vi "MaquinaDispensadora.vi"() -> ()   [LabVIEW 2020]
uses:
  Control 1.ctl
panel:
  out "Numeric":dbl
  out "Boolean":bool
  in  "stop":bool
  out "Cambio":dbl
  in  "Estado compra":string
  out "Total":dbl
  out "Precio":dbl
  in  "Moneda":cluster{"$ 10":bool, "$ 20":bool}
  in  "Productos":T1
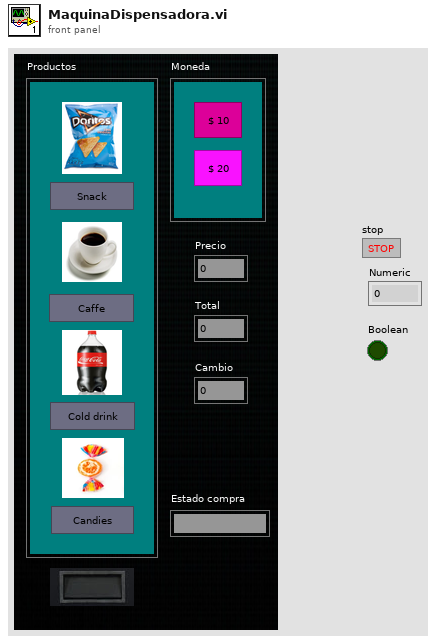
[diagram p1: front panel]
types:
  T1 = cluster{"Snack":bool, "Caffe":bool, " Cold drink":bool, "Candies":bool}
  T2 = typedef "Control 1.ctl" = enum16{"Return Change", "Selecto Product", "Add Money", "Waiting", "Start-UP", "Dispense Product"}
  T3 = cluster{"Cherry Rush":bool, "Lime Fizz":bool, "Orange Blast":bool, "Mr. Fizzle":bool}
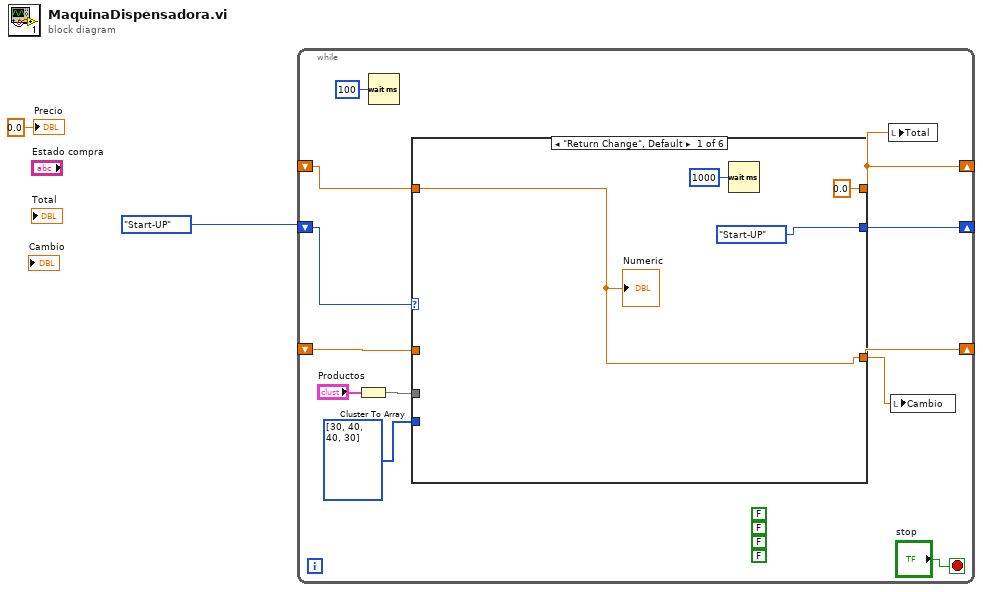
[diagram p0: block diagram]
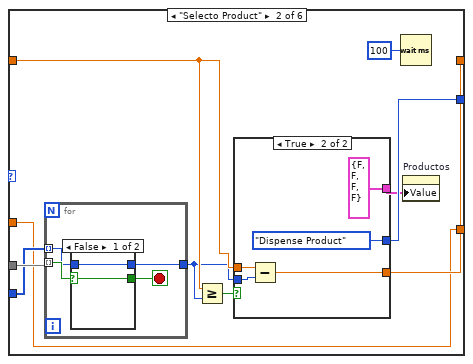
[diagram p2: hidden frame]
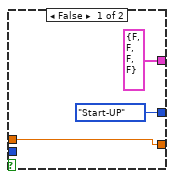
[diagram p3: hidden frame]
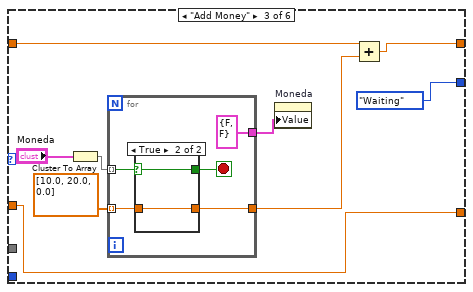
[diagram p5: hidden frame]
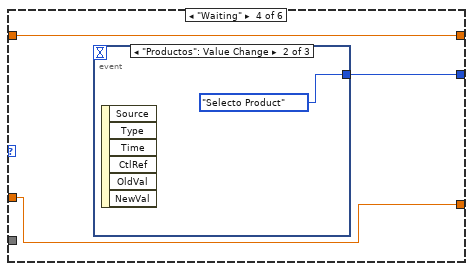
[diagram p7: hidden frame]
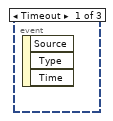
[diagram p8: hidden frame]
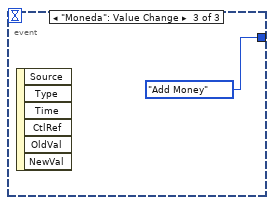
[diagram p9: hidden frame]
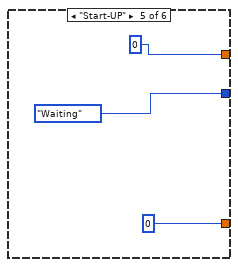
[diagram p10: hidden frame]
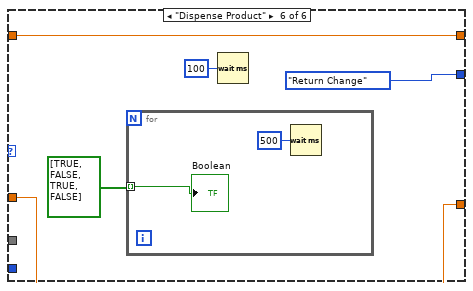
[diagram p11: hidden frame]
diagram:
  n1 = while {
    shift-right: [w9] -> _
    shift-left: Control_1."Start-UP" -> [w11]
    shift-right: [w5] -> _
    shift-left: _ -> [w6]
    shift-right: [w4] -> _
    shift-left: _ -> [w10]
    stop <- "stop" stop-if-true
    (unwired) FALSE ("Mr. Fizzle")
    (unwired) FALSE ("Orange Blast")
    (unwired) FALSE ("Lime Fizz")
    (unwired) FALSE ("Cherry Rush")
    n2 = Cluster To Array(cluster="Productos") -> (array=w8:bool[])
    n3 = Wait (ms)(milliseconds to wait=u32 100) -> ()  [unwired: 1 out]
    n4 = case shown="\"Return Change\", Default" w11 {
      tunnel: [0.0 w22 w48 w63 0 w71] -> w5
      tunnel: [w15 w18 w44 w64 0 w72] -> w4
      tunnel: w10 -> [_ w18 w44 w64 _ w72]
      tunnel: [Control_1."Start-UP" w21 Control_1."Waiting" w62 Control_1."Waiting" Control_1."Return Change"] -> w9
      tunnel: w8 -> [_ w27 _ _ _ _]
      tunnel: i32[] [30, 40, 40, 30] -> [_ w26 _ _ _ _]
      tunnel: w6 -> [w15 w24 w47 w63 _ w71]
      frame "Return Change", Default {
        n5 = Wait (ms)(milliseconds to wait=u32 1000) -> ()  [unwired: 1 out]
        "Numeric" <- w15
      }
      frame "Selecto Product" {
        n6 = for {
          tunnel: w27 -> [w39] mode=indexing
          tunnel: w26 -> [w37] mode=indexing
          tunnel: [w36] -> w23
          stop <- w38 stop-if-true
          n7 = case shown="False" w39 {
            selector: w39 -> [w41 w43]
            tunnel: [w41 w43] -> w38
            tunnel: w37 -> [w40 w42]
            tunnel: [w40 w42] -> w36
            frame False {
            }
            frame True {
            }
          }
        }
        n8 = Greater Or Equal?(x=w24, y=w23) -> (x >= y?=w25:bool)
        n9 = case shown="True" w25 {
          tunnel: w24 -> [w30 w35]
          tunnel: w23 -> [_ w34]
          tunnel: [w30 w33] -> w22
          tunnel: [Control_1."Start-UP" Control_1."Dispense Product"] -> w21
          tunnel: [T3 {"Cherry Rush"=FALSE, "Lime Fizz"=FALSE, "Orange Blast"=FALSE, "Mr. Fizzle"=FALSE} ("Choose from \nthese:") T3 {"Cherry Rush"=FALSE, "Lime Fizz"=FALSE, "Orange Blast"=FALSE, "Mr. Fizzle"=FALSE} ("Choose from \nthese:")] -> w20
          frame False {
          }
          frame True {
            n10 = Subtract(x=w35, y=w34) -> (x-y=w33:dbl)
          }
        }
        n11 = Wait (ms)(milliseconds to wait=u32 100) -> ()  [unwired: 1 out]
        n12 = property on="Productos" class="Clust (strict)"("Value"=w20) -> ()  [unwired: 2 in, 2 out]
      }
      frame "Add Money" {
        n13 = Cluster To Array(cluster="Moneda") -> (array=w51:bool[])
        n14 = for {
          tunnel: w51 -> [w57] mode=indexing
          tunnel: dbl[] [10.0, 20.0, 0.0] -> [w55] mode=indexing
          tunnel: [w54] -> w46
          tunnel: [cluster{"10 Cents":bool, "5 Cents":bool} {"10 Cents"=FALSE, "5 Cents"=FALSE} ("Insert Coins")] -> w49
          stop <- w56 stop-if-true
          n15 = case shown="True" w57 {
            selector: w57 -> [w59 w61]
            tunnel: [w59 w61] -> w56
            tunnel: w55 -> [w58 w60]
            tunnel: [w58 w60] -> w54
            frame False {
            }
            frame True {
            }
          }
        }
        n16 = property on="Moneda" class="Clust (strict)"("Value"=w49) -> ()  [unwired: 2 in, 2 out]
        n17 = Add(x=w47, y=w46) -> (x+y=w48:dbl)
      }
      frame "Waiting" {
        n18 = event shown="[1] \"Productos\": Value Change" {
          selector: _ -> [_ _ _]
          dyn-events: _ -> [_ _ _]
          timeout: _ -> [_ _ _]
          tunnel: [_ Control_1."Selecto Product" Control_1."Add Money"] -> w62
          event Timeout {
            n19 = event-data() -> ()  [unwired: 1 in, 3 out]
          }
          event "Productos": Value Change {
            n20 = event-data() -> ()  [unwired: 1 in, 6 out]
          }
          event "Moneda": Value Change {
            n21 = event-data() -> ()  [unwired: 1 in, 6 out]
          }
        }
      }
      frame "Start-UP" {
      }
      frame "Dispense Product" {
        n22 = for {
          tunnel: bool[] [TRUE, FALSE, TRUE, FALSE] -> [w76] mode=indexing
          n23 = Wait (ms)(milliseconds to wait=u32 500) -> ()  [unwired: 1 out]
          "Boolean" <- w76
        }
        n24 = Wait (ms)(milliseconds to wait=u32 100) -> ()  [unwired: 1 out]
      }
    }
    n25 = local write "Total"(w5) -> ()
    n26 = local write "Cambio"(w4) -> ()
  }
  "Precio" <- 0.0 ("Precio")
